vi "Pre Launch Init.vi"(11 "User Interface in":refnum<class "User Interface.lvclass">) -> (0 "error out":errorcluster, 3 "User Interface out":refnum<class "User Interface.lvclass">)   [LabVIEW 2015, in "User Interface.lvlib" / "User Interface.lvclass"]
doc: "(<B>Filename</B>: Actor Framework.lvlib:Actor.lvclass:Pre Launch Init.vi)\n\nDefines behavior that occurs after the Launch Nested Actor method is invoked but before the actor's Actor Core method begins running.\n\nBy default, this method does nothing. A descendant class may override it to define behavior."
uses:
  User Interface.lvclass
  <vilib>/ActorFramework/Actor/Actor.lvclass/Actor.ctl
  <vilib>/ActorFramework/Message Enqueuer/Message Enqueuer.lvclass/Message Enqueuer.ctl
  User Interface.lvclass/User Interface.ctl
  <vilib>/ActorFramework/Message Enqueuer/Enqueue.vi
  <vilib>/ActorFramework/Message Enqueuer/Init from Existing Queue.vi
  <vilib>/ActorFramework/Message Priority Queue/Priority Enqueue.vi
  User Interface Messages/Set Default Values Msg/Set Default Values Msg.lvclass
  <vilib>/ActorFramework/Message Enqueuer/Message Enqueuer.lvclass
  <vilib>/ActorFramework/Actor/Actor.lvclass
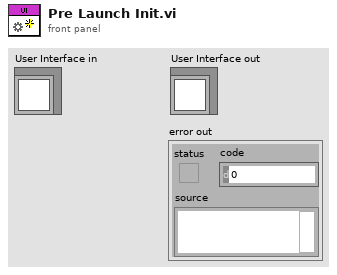
[diagram p1: front panel]
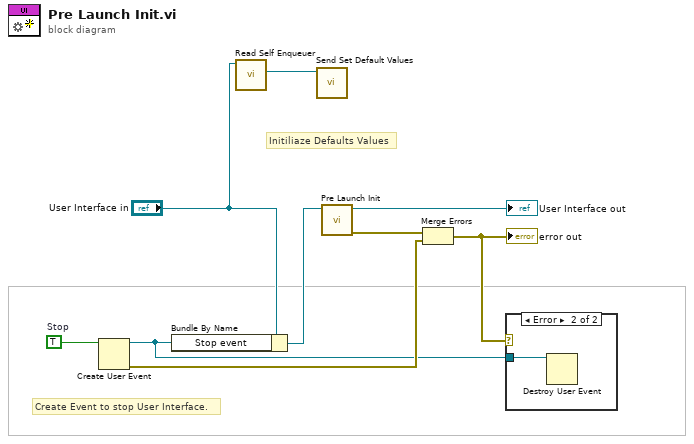
[diagram p0: block diagram]
diagram:
  w8 = TRUE  # Stop
  # "Create Event to stop User Interface."
  # "Initiliaze Defaults Values"
  n1 = Create User Event(user event datatype=w8) -> (user event=w3:refnum<user-event>, error out=w4:errorcluster)  [unwired: 1 in]
  n2 = Bundle By Name(cluster="User Interface in", "Stop event"=w3) -> (w7:refnum<class "User Interface.lvclass">)
  n3 = call <vilib>:"Read Self Enqueuer.vi"("Actor"="User Interface in") -> ("Self Enqueuer"=w1:refnum<class "Message Enqueuer.lvclass">)  [unwired: 10 in]
  n4 = call "Send Set Default Values.vi"("Message Enqueuer"=w1) -> ()  [unwired: 9 in, 2 out]
  n5 = call-parent "Pre Launch Init.vi"("Actor in"=w7) -> ("error out"=w6:errorcluster, "Actor out"=→"User Interface out":refnum<class "User Interface.lvclass">)  [unwired: 9 in]
  n6 = Merge Errors(w6, w4) -> (w5:errorcluster)
  "error out" <- w5
  n7 = case shown="Error" w5 {
    tunnel: w3 -> [_ w10]
    frame No Error {
    }
    frame Error {
      n8 = Destroy User Event(user event=w10) -> ()  [unwired: 1 in, 1 out]
    }
  }
